vi "RampDown.vi"(1 "Decrease per Cycle":dbl, 2 "Input":dbl) -> (0 "Output":dbl)   [LabVIEW 2020, in "TitanLib.lvlib"]
uses:
  TitanLib.lvlib
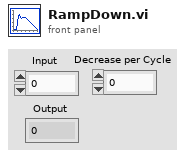
[diagram p1: front panel]
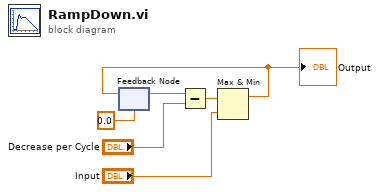
[diagram p0: block diagram]
diagram:
  n1 = feedback #1(0.0) -> (w3:dbl)
  n2 = Subtract(x=w3, y="Decrease per Cycle") -> (x-y=w4:dbl)
  n3 = Max & Min(x=w4, y="Input") -> (max(x,y)=w2:dbl)  [unwired: 1 out]
  "Output" <- w2
  n4 = feedback-in #1(w2) -> ()
